vi "constants.vi"(4 "DB connection file path in":path=path "") -> (0 "file path for Processed Signal .hdf5 files":path, 1 "DB connection file path":path=path "C:/Program Files (x86)/National Instruments/LabVIEW 2013/user.lib/Accelerator/User Interface/Database Connection.vi", 2 "Testing":bool=TRUE)   [LabVIEW 2013]
doc: "Detects if the computer is on a production computer or a test computer and ouputs paths to various useful locations based on whether or not it is testing."
uses:
  <userlib>/_OpenG.lib/file/file.llb/File Exists - Scalar__ogtk.vi
panel:
  # "If you are here because of error 8360:\n  1. Stop running all vis that are using this program. These include the batch processor, the live plot, BigAccDAQ, and several others.\n  1. Click on the folder symbol to the far right below.\n  2. Find and select the Database Connection vi. It should be in the user.lib folder under the version of LabVIEW displaying this program.\n  3. Run the program.\n  4. If successful, the program will display the new file path in \"DB connection file path\" below. If not, try again.\n  5. Right click on \"DB connection file path\" and select Data Operations>Make Current Value Default.\nClose this program when you are finished."
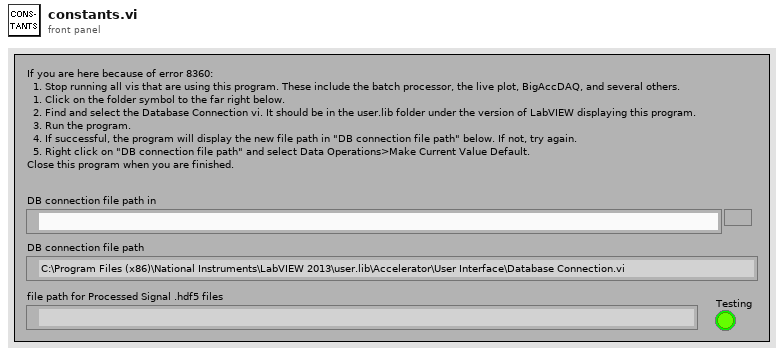
[diagram p1: front panel]
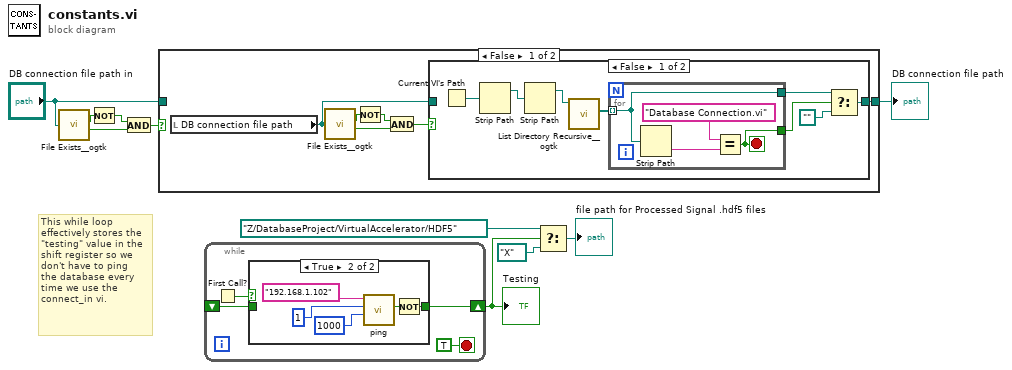
[diagram p0: block diagram]
diagram:
  # "This while loop\neffectively stores the\n\"testing\" value in the\nshift register so we\ndon't have to ping\nthe database every\ntime we use the\nconnect_in vi."
  n1 = call-poly <userlib>:"File Exists__ogtk.vi"("file path"="DB connection file path in") -> ("is directory"=w5:bool, "exists"=w6:bool)  [unwired: 6 in]
  n2 = Not(x=w5) -> (.not. x?=w4:bool)
  n3 = And(x=w4, y=w6) -> (x .and. y?=w3:bool)
  n4 = case shown="False" w3 {
    tunnel: [w13 w30] -> w2
    tunnel: "DB connection file path in" -> [_ w30]
    frame False {
      n5 = local read "DB connection file path"() -> (w11:path)
      n6 = call-poly <userlib>:"File Exists__ogtk.vi"("file path"=w11) -> ("is directory"=w15:bool, "exists"=w14:bool)  [unwired: 6 in]
      n7 = Not(x=w15) -> (.not. x?=w16:bool)
      n8 = And(x=w16, y=w14) -> (x .and. y?=w12:bool)
      n9 = case shown="False" w12 {
        tunnel: [w17 w29] -> w13
        tunnel: w11 -> [_ w29]
        frame False {
          n10 = Current VI's Path() -> (path=w24:path)
          n11 = Strip Path(path=w24) -> (stripped path=w22:path)  [unwired: 1 out]
          n12 = Strip Path(path=w22) -> (stripped path=w21:path)  [unwired: 1 out]
          n13 = call <userlib>:"List Directory Recursive__ogtk.vi"("Path"=w21) -> ("file paths"=w23:path[])  [unwired: 7 in, 3 out]
          n14 = for {
            tunnel: w23 -> [w28] mode=indexing
            tunnel: [w28] -> w20
            tunnel: [w25] -> w19
            stop <- w25 stop-if-true
            n15 = Strip Path(path=w28) -> (name=w27:string)  [unwired: 1 out]
            n16 = Equal?(x="Database Connection.vi", y=w27) -> (x = y?=w25:bool)
          }
          n17 = Select(t=w20, s=w19, f=path "") -> (s? t:f=w17:path)
        }
        frame True {
        }
      }
    }
    frame True {
    }
  }
  "DB connection file path" <- w2
  n18 = while {
    shift-right: [w34] -> w7
    shift-left: _ -> [w31]
    stop <- TRUE stop-if-true
    n19 = First Call?() -> (First Call?: T/F=w33:bool)
    n20 = case shown="True" w33 {
      tunnel: [w35 w36] -> w34
      tunnel: w31 -> [w35 _]
      frame False {
      }
      frame True {
        n21 = call <userlib>:"ping.vi"("timeout (ms)"=1000, "count"=1, "host"="192.168.1.102") -> ("found?"=w37:bool)  [unwired: 6 in, 2 out]
        n22 = Not(x=w37) -> (.not. x?=w36:bool)
      }
    }
  }
  "Testing" <- w7
  n23 = Select(t=path "Z:/DatabaseProject/VirtualAccelerator/HDF5", s=w7, f=path "X:/") -> (s? t:f=→"file path for Processed Signal .hdf5 files":path)
